vi "SystemMode.vi"(7 "Write?":bool, 11 "ModeInput":enum16{"Off", "Reading", "Writing"}(ring)) -> (3 "Mode":enum16{"Off", "Reading", "Writing"}(ring))   [LabVIEW 2010, in "Packet Recorder.lvlib"]
uses:
  Packet Recorder.lvlib
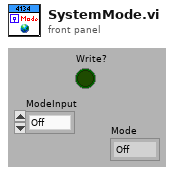
[diagram p1: front panel]
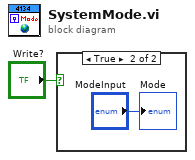
[diagram p0: block diagram]
diagram:
  n1 = case shown="True" "Write?" {
    frame False {
    }
    frame True {
      "Mode" <- "ModeInput"
    }
  }
